vi "StellarNet Calculate Wavelengths, ext precision.vi"(1 "C's":ext[](array[numeric])) -> (0 "Wavelengths":dbl[](array[numeric]))   [LabVIEW 2023]
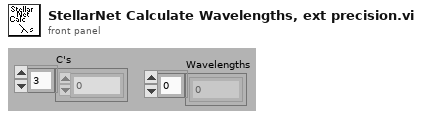
[diagram p1: front panel]
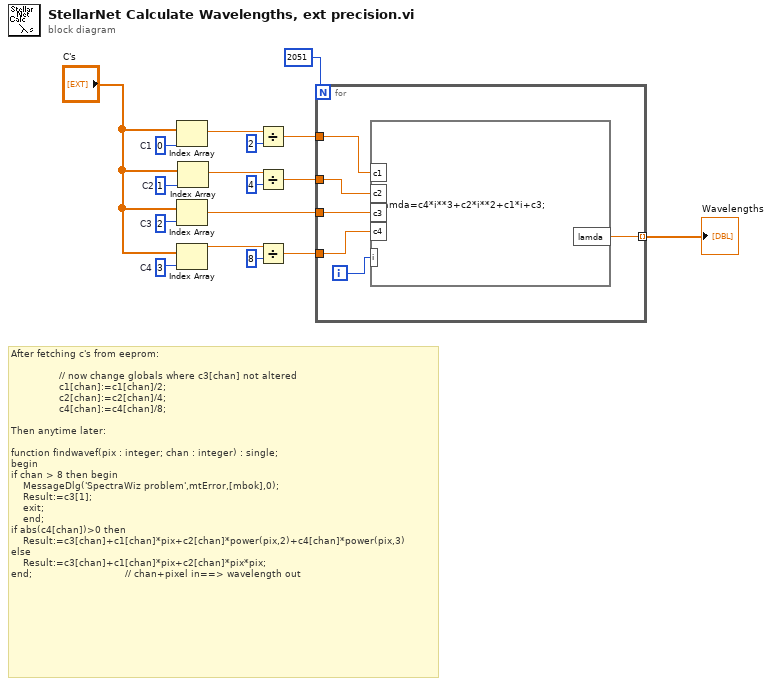
[diagram p0: block diagram]
diagram:
  w9 = 3  # C4
  w16 = 0  # C1
  w15 = 2  # C3
  w17 = 1  # C2
  # "After fetching c's from eeprom:\n\n                // now change globals where c3[chan] not altered\n                c1[chan]:=c1[chan]/2;\n                c2[chan]:=c2[chan]/4;\n                c4[chan]:=c4[chan]/8;\n\nThen anytime later:\n\nfunction findwavef(pix : integer; chan : integer) : single;\nbegin\nif chan > 8 then begin\n    MessageDlg('SpectraWiz problem',mtError,[mbok],0);\n    Result:=c3[1];\n    exit;\n    end;\nif abs(c4[chan])>0 then\n    Result:=c3[chan]+c1[chan]*pix+c2[chan]*power(pix,2)+c4[chan]*power(pix,3)\nelse\n    Result:=c3[chan]+c1[chan]*pix+c2[chan]*pix*pix;\nend;                               // chan+pixel in==> wavelength out"
  n1 = Index Array(array="C's", index=w16) -> (element=w12:ext)
  n2 = Index Array(array="C's", index=w15) -> (element=w5:ext)
  n3 = Index Array(array="C's", index=w9) -> (element=w1:ext)
  n4 = Index Array(array="C's", index=w17) -> (element=w10:ext)
  n5 = Divide(x=w12, y=u8 2) -> (x/y=w7:ext)
  n6 = Divide(x=w10, y=u8 4) -> (x/y=w6:ext)
  n7 = Divide(x=w1, y=u8 8) -> (x/y=w2:ext)
  n8 = for {
    N: 2051 -> [_]
    tunnel: w7 -> [w22]
    tunnel: w6 -> [w21]
    tunnel: w5 -> [w20]
    tunnel: w2 -> [w19]
    tunnel: [w18] -> w4 mode=indexing
    i -> [w23]
    n9 = formula code="lamda=c4*i**3+c2*i**2+c1*i+c3;"("c2"=w21, "c3"=w20, "c4"=w19, "i"=w23, "c1"=w22) -> ("lamda"=w18:dbl)
  }
  "Wavelengths" <- w4
